vi "Plotter Selector.vi"(10 "Ring Selector":u16, 11 "CAR DATA":T1) -> (0 "Y Label":string, 1 "Plot Output":cluster{"Time":dbl[], "yi":dbl[]}, 2 "Y Minimum":dbl, 3 "Y Maximum":dbl)   [LabVIEW 2014]
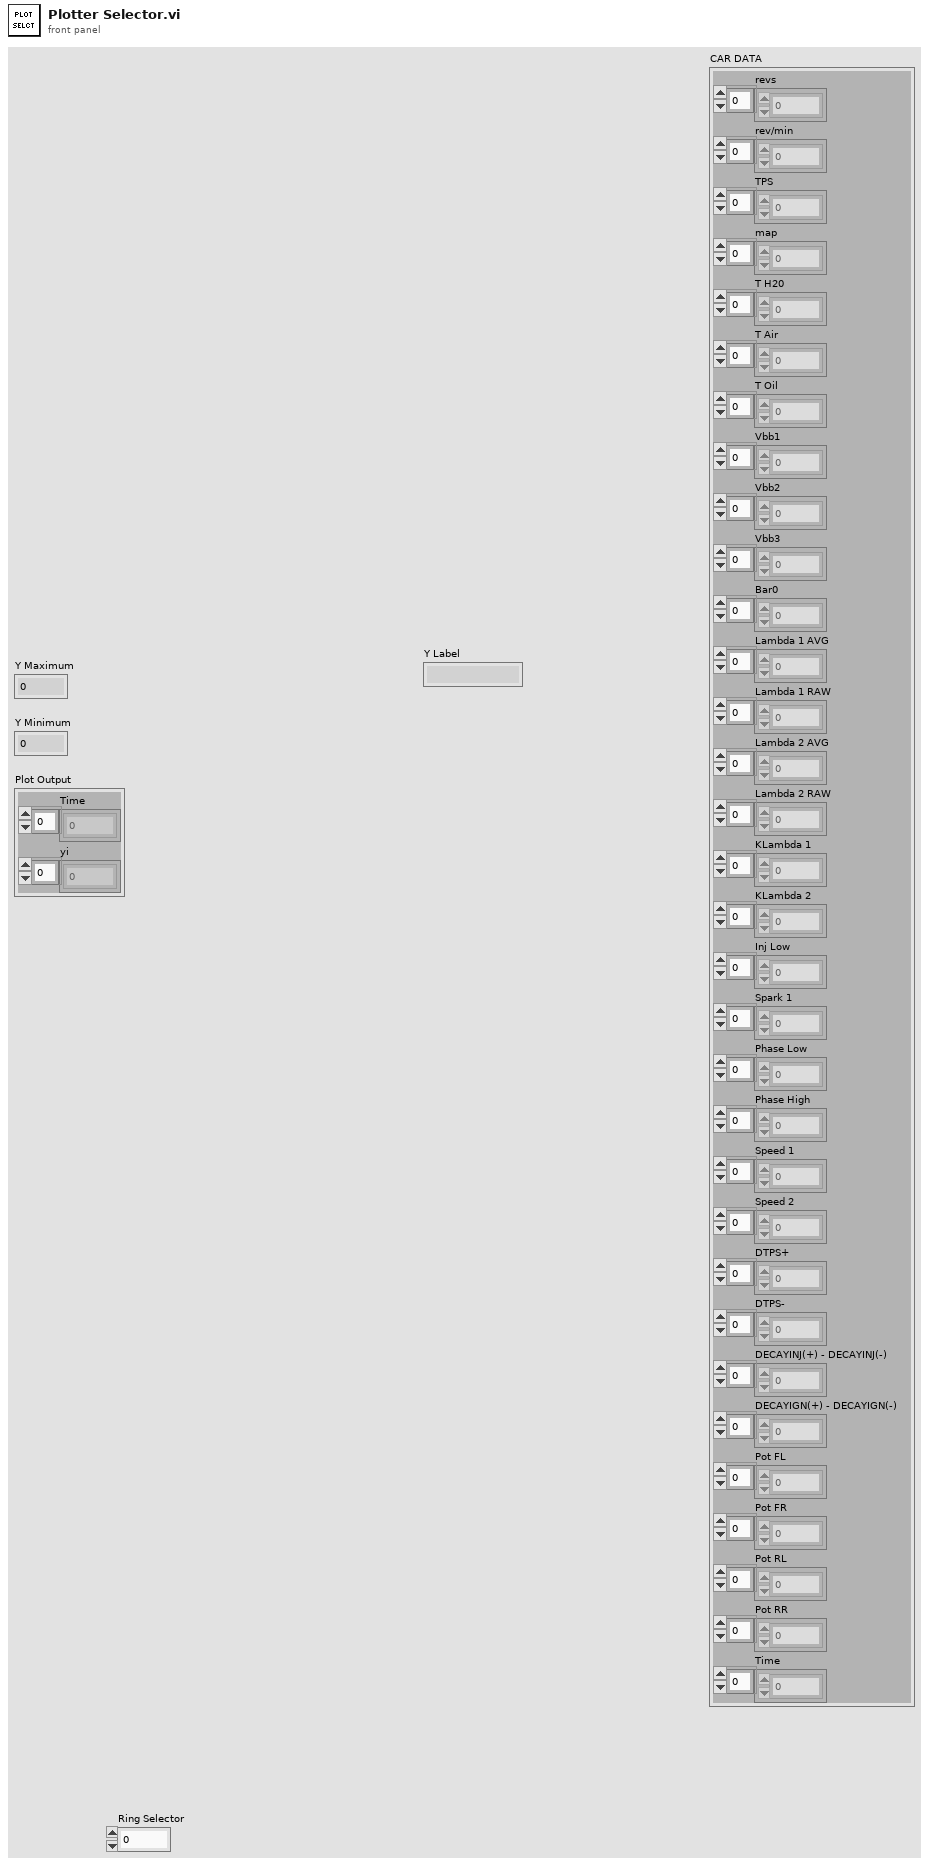
[diagram p1: front panel]
types:
  T1 = cluster{"revs":dbl[], "rev/min":dbl[], "TPS":dbl[], "map":dbl[], "T H20":dbl[], "T Air":dbl[], "T Oil":dbl[], "Vbb1":dbl[], "Vbb2":dbl[], "Vbb3":dbl[], "Bar0":dbl[], "Lambda 1 AVG":dbl[], "Lambda 1 RAW":dbl[], "Lambda 2 AVG":dbl[], "Lambda 2 RAW":dbl[], "KLambda 1":dbl[], "KLambda 2":dbl[], "Inj Low":dbl[], "Spark 1":dbl[], "Phase Low":dbl[], "Phase High":dbl[], "Speed 1":dbl[], "Speed 2":dbl[], "DTPS+":dbl[], "DTPS-":dbl[], "DECAYINJ(+) - DECAYINJ(-)":dbl[], "DECAYIGN(+) - DECAYIGN(-)":dbl[], "Pot FL":dbl[], "Pot FR":dbl[], "Pot RL":dbl[], "Pot RR":dbl[], "Time":dbl[]}
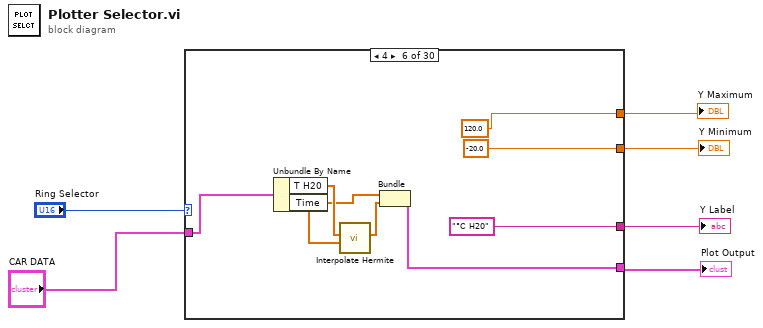
[diagram p0: block diagram]
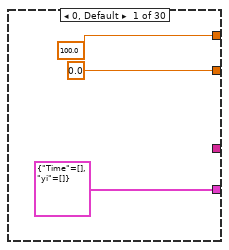
[diagram p2: hidden frame]
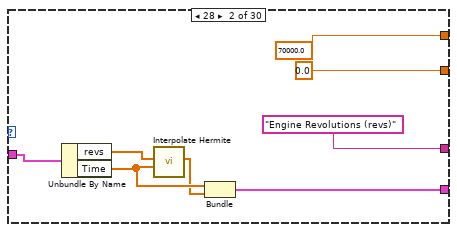
[diagram p3: hidden frame]
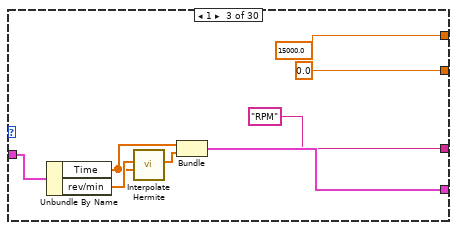
[diagram p4: hidden frame]
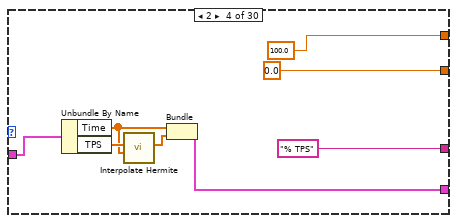
[diagram p5: hidden frame]
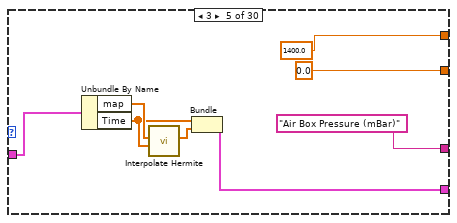
[diagram p6: hidden frame]
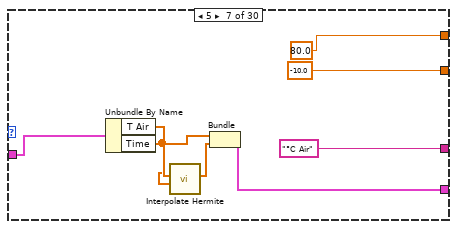
[diagram p7: hidden frame]
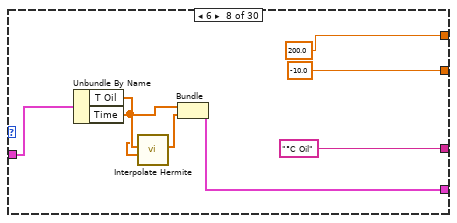
[diagram p8: hidden frame]
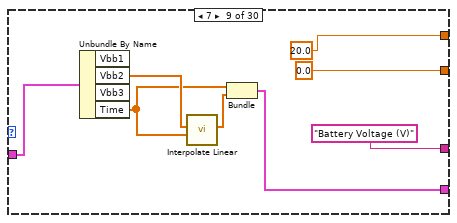
[diagram p9: hidden frame]
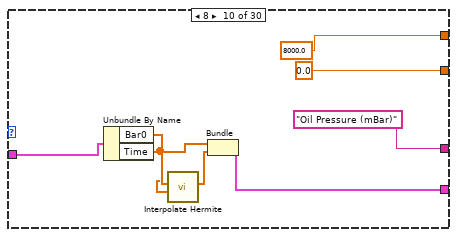
[diagram p10: hidden frame]
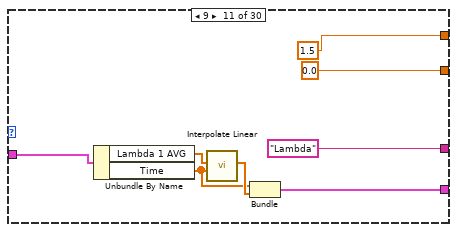
[diagram p11: hidden frame]
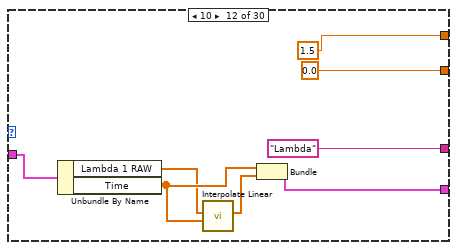
[diagram p12: hidden frame]
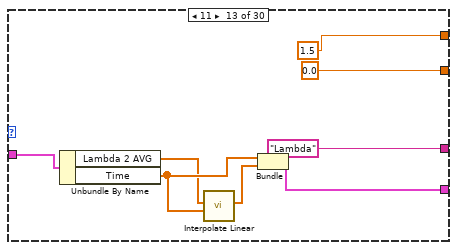
[diagram p13: hidden frame]
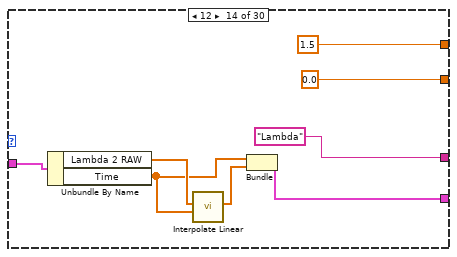
[diagram p14: hidden frame]
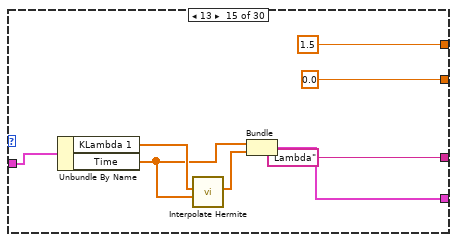
[diagram p15: hidden frame]
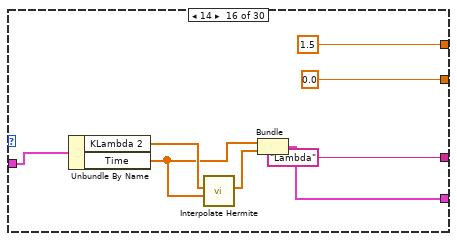
[diagram p16: hidden frame]
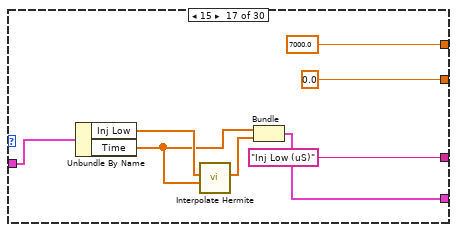
[diagram p17: hidden frame]
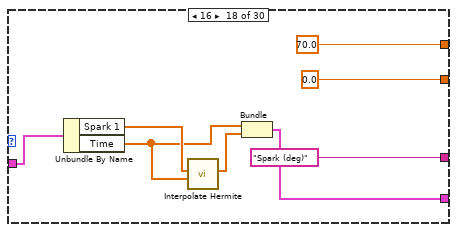
[diagram p18: hidden frame]
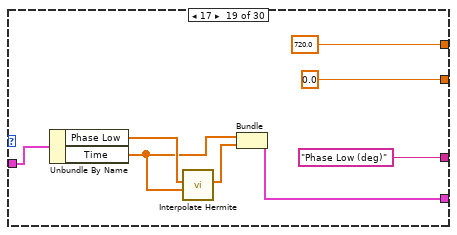
[diagram p19: hidden frame]
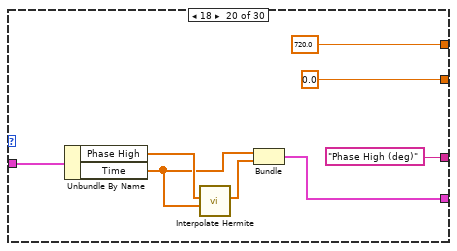
[diagram p20: hidden frame]
diagram:
  n1 = case shown="4" "Ring Selector" {
    tunnel: [cluster{"Time":dbl[], "yi":dbl[]} {"Time"=[], "yi"=[]} w14 w23 w31 w39 w47 w55 w63 w66 w79 w88 w94 w102 w110 w118 w126 w134 w142 w150 w158 w167 w174 w182 w187 w192 w199 w205 w213 w221 w228] -> w6
    tunnel: [0.0 ("Y Scale.Range:Maximum") 0.0 ("Y Scale.Range:Maximum") 0.0 ("Y Scale.Range:Maximum") 0.0 ("Y Scale.Range:Maximum") 0.0 ("Y Scale.Range:Maximum") -20.0 ("Y Scale.Range:Maximum") -10.0 ("Y Scale.Range:Maximum") -10.0 ("Y Scale.Range:Maximum") 0.0 ("Y Scale.Range:Maximum") 0.0 ("Y Scale.Range:Maximum") 0.0 ("Y Scale.Range:Maximum") 0.0 ("Y Scale.Range:Maximum") 0.0 ("Y Scale.Range:Maximum") 0.0 ("Y Scale.Range:Maximum") 0.0 ("Y Scale.Range:Maximum") 0.0 ("Y Scale.Range:Maximum") 0.0 ("Y Scale.Range:Maximum") 0.0 ("Y Scale.Range:Maximum") 0.0 ("Y Scale.Range:Maximum") 0.0 ("Y Scale.Range:Maximum") 0.0 ("Y Scale.Range:Maximum") 0.0 ("Y Scale.Range:Maximum") 0.0 ("Y Scale.Range:Maximum") _ _ 0.0 ("Y Scale.Range:Maximum") 0.0 ("Y Scale.Range:Maximum") 0.0 ("Y Scale.Range:Maximum") 0.0 ("Y Scale.Range:Maximum") 0.0 ("Y Scale.Range:Maximum")] -> w4
    tunnel: [100.0 ("Y Scale.Range:Maximum") 70000.0 ("Y Scale.Range:Maximum") 15000.0 ("Y Scale.Range:Maximum") 100.0 ("Y Scale.Range:Maximum") 1400.0 ("Y Scale.Range:Maximum") 120.0 ("Y Scale.Range:Maximum") 80.0 ("Y Scale.Range:Maximum") 200.0 ("Y Scale.Range:Maximum") 20.0 ("Y Scale.Range:Maximum") 8000.0 ("Y Scale.Range:Maximum") 1.5 ("Y Scale.Range:Maximum") 1.5 ("Y Scale.Range:Maximum") 1.5 ("Y Scale.Range:Maximum") 1.5 ("Y Scale.Range:Maximum") 1.5 ("Y Scale.Range:Maximum") 1.5 ("Y Scale.Range:Maximum") 7000.0 ("Y Scale.Range:Maximum") 70.0 ("Y Scale.Range:Maximum") 720.0 ("Y Scale.Range:Maximum") 720.0 ("Y Scale.Range:Maximum") 300.0 ("Y Scale.Range:Maximum") 100.0 ("Y Scale.Range:Maximum") 100.0 ("Y Scale.Range:Maximum") _ _ 6.0 ("Y Scale.Range:Maximum") 6.0 ("Y Scale.Range:Maximum") 6.0 ("Y Scale.Range:Maximum") 6.0 ("Y Scale.Range:Maximum") 10.0 ("Y Scale.Range:Maximum")] -> w5
    tunnel: [_ "Engine Revolutions (revs)" "RPM" "% TPS" "Air Box Pressure (mBar)" "°C H20" "°C Air" "°C Oil" "Battery Voltage (V)" "Oil Pressure (mBar)" "Lambda" "Lambda" "Lambda" "Lambda" "Lambda" "Lambda" "Inj Low (uS)" "Spark (deg)" "Phase Low (deg)" "Phase High (deg)" "Speed (km/h)" "% DTPS+" "% DTPS -" _ _ "Potentiometer excursion (cm)" "Potentiometer excursion (cm)" "Potentiometer excursion (cm)" "Potentiometer excursion (cm)" "Gear"] -> w2
    tunnel: "CAR DATA" -> [_ w10 w18 w26 w34 w42 w50 w58 w68 w74 w82 w90 w98 w106 w114 w122 w130 w138 w146 w154 w163 w170 w178 w186 w191 w203 w208 w216 w224 w238]
    frame 0, Default {
    }
    frame 28 {
      n2 = Unbundle By Name(w10) -> ("revs"=w17:dbl[], "Time"=w16:dbl[])
      n3 = call "Interpolate Hermite.vi"("X in"=w16, "Y in"=w17) -> ("yi"=w15:dbl[])  [unwired: 9 in]
      n4 = Bundle("Time"=w16, "yi"=w15) -> (w14:cluster{"Time":dbl[], "yi":dbl[]})  [unwired: 1 in]
    }
    frame 1 {
      n5 = Unbundle By Name(w18) -> ("Time"=w22:dbl[], "rev/min"=w25:dbl[])
      n6 = call "Interpolate Hermite.vi"("X in"=w22, "Y in"=w25) -> ("yi"=w24:dbl[])  [unwired: 9 in]
      n7 = Bundle("Time"=w22, "yi"=w24) -> (w23:cluster{"Time":dbl[], "yi":dbl[]})  [unwired: 1 in]
    }
    frame 2 {
      n8 = Unbundle By Name(w26) -> ("Time"=w28:dbl[], "TPS"=w33:dbl[])
      n9 = call "Interpolate Hermite.vi"("X in"=w28, "Y in"=w33) -> ("yi"=w32:dbl[])  [unwired: 9 in]
      n10 = Bundle("Time"=w28, "yi"=w32) -> (w31:cluster{"Time":dbl[], "yi":dbl[]})  [unwired: 1 in]
    }
    frame 3 {
      n11 = Unbundle By Name(w34) -> ("map"=w41:dbl[], "Time"=w38:dbl[])
      n12 = call "Interpolate Hermite.vi"("X in"=w38, "Y in"=w41) -> ("yi"=w40:dbl[])  [unwired: 9 in]
      n13 = Bundle("Time"=w38, "yi"=w40) -> (w39:cluster{"Time":dbl[], "yi":dbl[]})  [unwired: 1 in]
    }
    frame 4 {
      n14 = Unbundle By Name(w42) -> ("T H20"=w49:dbl[], "Time"=w44:dbl[])
      n15 = call "Interpolate Hermite.vi"("X in"=w44, "Y in"=w49) -> ("yi"=w48:dbl[])  [unwired: 9 in]
      n16 = Bundle("Time"=w44, "yi"=w48) -> (w47:cluster{"Time":dbl[], "yi":dbl[]})  [unwired: 1 in]
    }
    frame 5 {
      n17 = Unbundle By Name(w50) -> ("T Air"=w57:dbl[], "Time"=w52:dbl[])
      n18 = call "Interpolate Hermite.vi"("X in"=w52, "Y in"=w57) -> ("yi"=w56:dbl[])  [unwired: 9 in]
      n19 = Bundle("Time"=w52, "yi"=w56) -> (w55:cluster{"Time":dbl[], "yi":dbl[]})  [unwired: 1 in]
    }
    frame 6 {
      n20 = Unbundle By Name(w58) -> ("T Oil"=w65:dbl[], "Time"=w62:dbl[])
      n21 = call "Interpolate Hermite.vi"("X in"=w62, "Y in"=w65) -> ("yi"=w64:dbl[])  [unwired: 9 in]
      n22 = Bundle("Time"=w62, "yi"=w64) -> (w63:cluster{"Time":dbl[], "yi":dbl[]})  [unwired: 1 in]
    }
    frame 7 {
      n23 = Unbundle By Name(w68) -> ("Vbb2"=w70:dbl[], "Time"=w67:dbl[])  [unwired: 2 out]
      n24 = call "Interpolate Linear.vi"("X in"=w67, "Y in"=w70) -> ("yi"=w73:dbl[])  [unwired: 9 in]
      n25 = Bundle("Time"=w67, "yi"=w73) -> (w66:cluster{"Time":dbl[], "yi":dbl[]})  [unwired: 1 in]
    }
    frame 8 {
      n26 = Unbundle By Name(w74) -> ("Bar0"=w80:dbl[], "Time"=w78:dbl[])
      n27 = call "Interpolate Hermite.vi"("X in"=w78, "Y in"=w80) -> ("yi"=w81:dbl[])  [unwired: 9 in]
      n28 = Bundle("Time"=w78, "yi"=w81) -> (w79:cluster{"Time":dbl[], "yi":dbl[]})  [unwired: 1 in]
    }
    frame 9 {
      n29 = Unbundle By Name(w82) -> ("Lambda 1 AVG"=w89:dbl[], "Time"=w86:dbl[])
      n30 = call "Interpolate Linear.vi"("X in"=w86, "Y in"=w89) -> ("yi"=w87:dbl[])  [unwired: 9 in]
      n31 = Bundle("Time"=w86, "yi"=w87) -> (w88:cluster{"Time":dbl[], "yi":dbl[]})  [unwired: 1 in]
    }
    frame 10 {
      n32 = Unbundle By Name(w90) -> ("Lambda 1 RAW"=w95:dbl[], "Time"=w97:dbl[])
      n33 = call "Interpolate Linear.vi"("X in"=w97, "Y in"=w95) -> ("yi"=w96:dbl[])  [unwired: 9 in]
      n34 = Bundle("Time"=w97, "yi"=w96) -> (w94:cluster{"Time":dbl[], "yi":dbl[]})  [unwired: 1 in]
    }
    frame 11 {
      n35 = Unbundle By Name(w98) -> ("Lambda 2 AVG"=w103:dbl[], "Time"=w105:dbl[])
      n36 = call "Interpolate Linear.vi"("X in"=w105, "Y in"=w103) -> ("yi"=w104:dbl[])  [unwired: 9 in]
      n37 = Bundle("Time"=w105, "yi"=w104) -> (w102:cluster{"Time":dbl[], "yi":dbl[]})  [unwired: 1 in]
    }
    frame 12 {
      n38 = Unbundle By Name(w106) -> ("Lambda 2 RAW"=w113:dbl[], "Time"=w111:dbl[])
      n39 = call "Interpolate Linear.vi"("X in"=w111, "Y in"=w113) -> ("yi"=w112:dbl[])  [unwired: 9 in]
      n40 = Bundle("Time"=w111, "yi"=w112) -> (w110:cluster{"Time":dbl[], "yi":dbl[]})  [unwired: 1 in]
    }
    frame 13 {
      n41 = Unbundle By Name(w114) -> ("KLambda 1"=w121:dbl[], "Time"=w119:dbl[])
      n42 = call "Interpolate Hermite.vi"("X in"=w119, "Y in"=w121) -> ("yi"=w120:dbl[])  [unwired: 9 in]
      n43 = Bundle("Time"=w119, "yi"=w120) -> (w118:cluster{"Time":dbl[], "yi":dbl[]})  [unwired: 1 in]
    }
    frame 14 {
      n44 = Unbundle By Name(w122) -> ("KLambda 2"=w129:dbl[], "Time"=w127:dbl[])
      n45 = call "Interpolate Hermite.vi"("X in"=w127, "Y in"=w129) -> ("yi"=w128:dbl[])  [unwired: 9 in]
      n46 = Bundle("Time"=w127, "yi"=w128) -> (w126:cluster{"Time":dbl[], "yi":dbl[]})  [unwired: 1 in]
    }
    frame 15 {
      n47 = Unbundle By Name(w130) -> ("Inj Low"=w137:dbl[], "Time"=w135:dbl[])
      n48 = call "Interpolate Hermite.vi"("X in"=w135, "Y in"=w137) -> ("yi"=w136:dbl[])  [unwired: 9 in]
      n49 = Bundle("Time"=w135, "yi"=w136) -> (w134:cluster{"Time":dbl[], "yi":dbl[]})  [unwired: 1 in]
    }
    frame 16 {
      n50 = Unbundle By Name(w138) -> ("Spark 1"=w145:dbl[], "Time"=w143:dbl[])
      n51 = call "Interpolate Hermite.vi"("X in"=w143, "Y in"=w145) -> ("yi"=w144:dbl[])  [unwired: 9 in]
      n52 = Bundle("Time"=w143, "yi"=w144) -> (w142:cluster{"Time":dbl[], "yi":dbl[]})  [unwired: 1 in]
    }
    frame 17 {
      n53 = Unbundle By Name(w146) -> ("Phase Low"=w153:dbl[], "Time"=w151:dbl[])
      n54 = call "Interpolate Hermite.vi"("X in"=w151, "Y in"=w153) -> ("yi"=w152:dbl[])  [unwired: 9 in]
      n55 = Bundle("Time"=w151, "yi"=w152) -> (w150:cluster{"Time":dbl[], "yi":dbl[]})  [unwired: 1 in]
    }
    frame 18 {
      n56 = Unbundle By Name(w154) -> ("Phase High"=w161:dbl[], "Time"=w159:dbl[])
      n57 = call "Interpolate Hermite.vi"("X in"=w159, "Y in"=w161) -> ("yi"=w160:dbl[])  [unwired: 9 in]
      n58 = Bundle("Time"=w159, "yi"=w160) -> (w158:cluster{"Time":dbl[], "yi":dbl[]})  [unwired: 1 in]
    }
    frame 19 {
      n59 = Unbundle By Name(w163) -> ("Speed 1"=w162:dbl[], "Time"=w168:dbl[])  [unwired: 1 out]
      n60 = call "Interpolate Hermite.vi"("X in"=w168, "Y in"=w162) -> ("yi"=w169:dbl[])  [unwired: 9 in]
      n61 = Bundle("Time"=w168, "yi"=w169) -> (w167:cluster{"Time":dbl[], "yi":dbl[]})  [unwired: 1 in]
    }
    frame 20 {
      n62 = Unbundle By Name(w170) -> ("DTPS+"=w177:dbl[], "Time"=w175:dbl[])
      n63 = call "Interpolate Hermite.vi"("X in"=w175, "Y in"=w177) -> ("yi"=w176:dbl[])  [unwired: 9 in]
      n64 = Bundle("Time"=w175, "yi"=w176) -> (w174:cluster{"Time":dbl[], "yi":dbl[]})  [unwired: 1 in]
    }
    frame 21 {
      n65 = Unbundle By Name(w178) -> ("DTPS-"=w185:dbl[], "Time"=w183:dbl[])
      n66 = call "Interpolate Hermite.vi"("X in"=w183, "Y in"=w185) -> ("yi"=w184:dbl[])  [unwired: 9 in]
      n67 = Bundle("Time"=w183, "yi"=w184) -> (w182:cluster{"Time":dbl[], "yi":dbl[]})  [unwired: 1 in]
    }
    frame 22 {
      n68 = Unbundle By Name(w186) -> ("DECAYINJ(+) - DECAYINJ(-)"=w190:dbl[], "Time"=w188:dbl[])
      n69 = call "Interpolate Hermite.vi"("X in"=w188, "Y in"=w190) -> ("yi"=w189:dbl[])  [unwired: 9 in]
      n70 = Bundle("Time"=w188, "yi"=w189) -> (w187:cluster{"Time":dbl[], "yi":dbl[]})  [unwired: 1 in]
    }
    frame 23 {
      n71 = Unbundle By Name(w191) -> ("DECAYIGN(+) - DECAYIGN(-)"=w195:dbl[], "Time"=w193:dbl[])
      n72 = call "Interpolate Hermite.vi"("X in"=w193, "Y in"=w195) -> ("yi"=w194:dbl[])  [unwired: 9 in]
      n73 = Bundle("Time"=w193, "yi"=w194) -> (w192:cluster{"Time":dbl[], "yi":dbl[]})  [unwired: 1 in]
    }
    frame 24 {
      n74 = Unbundle By Name(w203) -> ("Pot FL"=w202:dbl[], "Time"=w201:dbl[])
      n75 = call "Interpolate Hermite.vi"("X in"=w201, "Y in"=w202) -> ("yi"=w200:dbl[])  [unwired: 9 in]
      n76 = Bundle("Time"=w201, "yi"=w200) -> (w199:cluster{"Time":dbl[], "yi":dbl[]})  [unwired: 1 in]
    }
    frame 25 {
      n77 = Unbundle By Name(w208) -> ("Pot FR"=w211:dbl[], "Time"=w210:dbl[])
      n78 = call "Interpolate Hermite.vi"("X in"=w210, "Y in"=w211) -> ("yi"=w209:dbl[])  [unwired: 9 in]
      n79 = Bundle("Time"=w210, "yi"=w209) -> (w205:cluster{"Time":dbl[], "yi":dbl[]})  [unwired: 1 in]
    }
    frame 26 {
      n80 = Unbundle By Name(w216) -> ("Pot RL"=w219:dbl[], "Time"=w218:dbl[])
      n81 = call "Interpolate Hermite.vi"("X in"=w218, "Y in"=w219) -> ("yi"=w217:dbl[])  [unwired: 9 in]
      n82 = Bundle("Time"=w218, "yi"=w217) -> (w213:cluster{"Time":dbl[], "yi":dbl[]})  [unwired: 1 in]
    }
    frame 27 {
      n83 = Unbundle By Name(w224) -> ("Pot RR"=w227:dbl[], "Time"=w226:dbl[])
      n84 = call "Interpolate Hermite.vi"("X in"=w226, "Y in"=w227) -> ("yi"=w225:dbl[])  [unwired: 9 in]
      n85 = Bundle("Time"=w226, "yi"=w225) -> (w221:cluster{"Time":dbl[], "yi":dbl[]})  [unwired: 1 in]
    }
    frame 29 {
      n86 = Unbundle By Name(w238) -> ("rev/min"=w234:dbl[], "Speed 1"=w233:dbl[], "Time"=w229:dbl[])
      n87 = call "Interpolate Linear.vi"("X in"=w229, "Y in"=w234) -> ("yi"=w231:dbl[])  [unwired: 9 in]
      n88 = call "Interpolate Linear.vi"("X in"=w229, "Y in"=w233) -> ("yi"=w232:dbl[])  [unwired: 9 in]
      n89 = Divide(x=w232, y=w231) -> (x/y=w230:dbl[])
      n90 = Bundle("Time"=w229, w230) -> (w228:cluster{"Time":dbl[], dbl[]})  [unwired: 1 in]
    }
  }
  "Plot Output" <- w6
  "Y Maximum" <- w5
  "Y Minimum" <- w4
  "Y Label" <- w2
